vi "Cruft Dialog.vi"(11 "Path":path) -> (3 "Result":enum16{"Add", "Ignore", "Abort"}(ring))   [LabVIEW 2024]
panel:
  in  "Abort":bool
  out "Prompt":string
  in  "Ignore":bool
  in  "Add":bool
  out "Image":picture
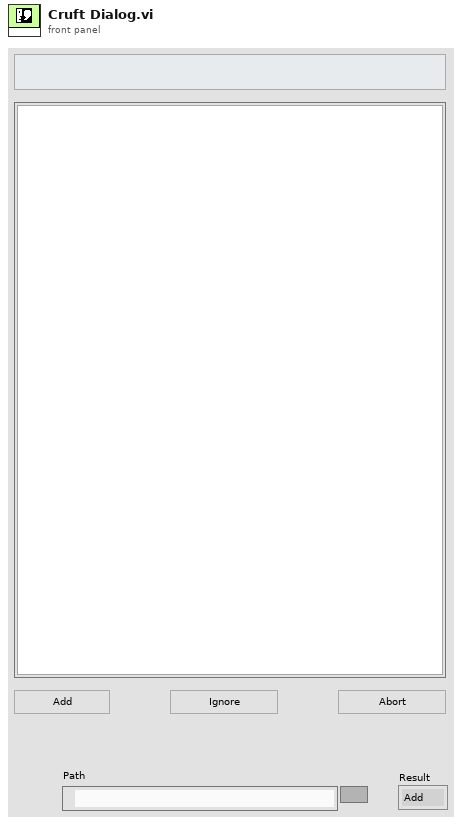
[diagram p1: front panel]
types:
  T1 = typedef "LVBoundsTypeDef.ctl" = cluster{"Width":u32, "Height":u32}
  T2 = typedef "imagedata.ctl" = cluster{"image type":i32, "image depth":i32, "image":u8[], "mask":u8[], "colors":u32[], "Rectangle":cluster{"left":i16, "top":i16, "right":i16, "bottom":i16}}
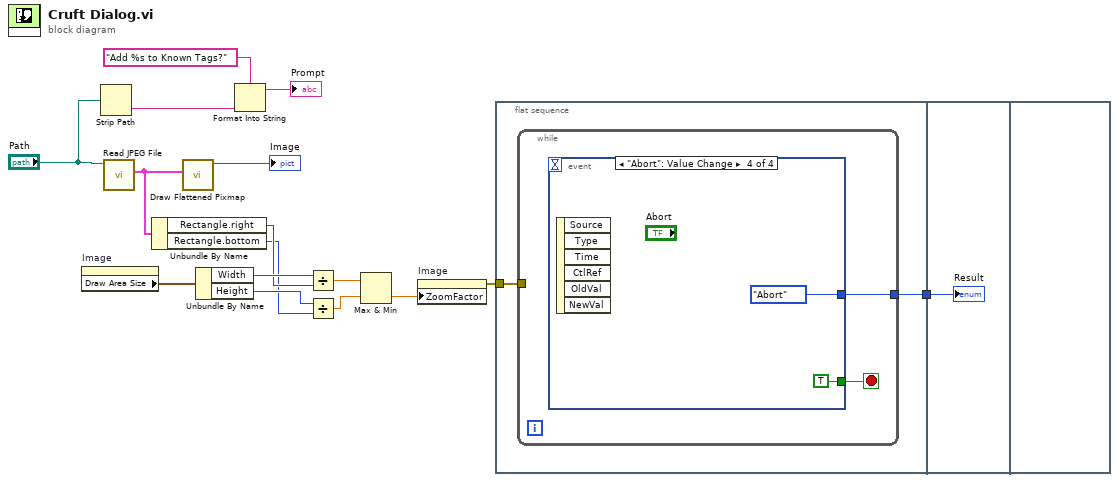
[diagram p0: block diagram]
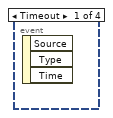
[diagram p2: hidden frame]
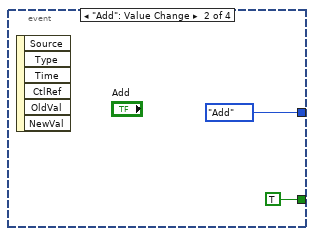
[diagram p3: hidden frame]
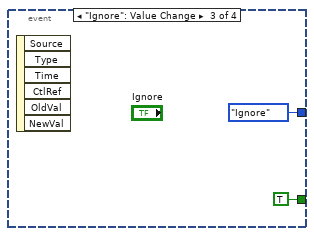
[diagram p4: hidden frame]
diagram:
  n1 = property on="Image" class="Pict"() -> ("Draw Area Size"=w15:T1)  [unwired: 2 in, 2 out]
  n2 = Strip Path(path="Path") -> (name=w3:string)  [unwired: 1 out]
  n3 = call <vilib>:"Read JPEG File.vi"("path to JPEG file"="Path") -> ("image data"=w14:T2)  [unwired: 8 in, 2 out]
  n4 = Unbundle By Name(w14) -> ("Rectangle.right"=w11:i16, "Rectangle.bottom"=w10:i16)
  n5 = call <vilib>:"Draw Flattened Pixmap.vi"("image data"=w14) -> ("new picture"=→"Image":picture)  [unwired: 8 in]
  n6 = Unbundle By Name(w15) -> ("Width"=w13:u32, "Height"=w12:u32)
  n7 = Format Into String(format string="Add %s to Known Tags?", w3) -> (resulting string=→"Prompt":string)  [unwired: 2 in, 1 out]
  n8 = Divide(x=w13, y=w11) -> (x/y=w9:dbl)
  n9 = Divide(x=w12, y=w10) -> (x/y=w8:dbl)
  n10 = Max & Min(x=w9, y=w8) -> (min(x,y)=w7:dbl)  [unwired: 1 out]
  n11 = property on="Image" class="Pict"("ZoomFactor"=w7) -> (error out=w6:errorcluster)  [unwired: 2 in, 1 out]
  n12 = flat-sequence {
    tunnel: w6 -> [w18]
    tunnel: [w17] -> w1
    tunnel: w1 -> [w27]
    frame #0 {
      n13 = while {
        tunnel: w18 -> [_]
        tunnel: [w20] -> w17
        stop <- w19 stop-if-true
        n14 = event shown="[3] \"Abort\": Value Change" {
          selector: _ -> [_ _ _ _]
          dyn-events: _ -> [_ _ _ _]
          timeout: _ -> [_ _ _ _]
          tunnel: [_ enum16{"Add", "Ignore", "Abort"}."Add" ("Result") enum16{"Add", "Ignore", "Abort"}."Ignore" ("Result") enum16{"Add", "Ignore", "Abort"}."Abort" ("Result")] -> w20
          tunnel: [_ TRUE TRUE TRUE] -> w19
          event Timeout {
            n15 = event-data() -> ()  [unwired: 1 in, 3 out]
          }
          event "Add": Value Change {
            n16 = event-data() -> ()  [unwired: 1 in, 6 out]
          }
          event "Ignore": Value Change {
            n17 = event-data() -> ()  [unwired: 1 in, 6 out]
          }
          event "Abort": Value Change {
            n18 = event-data() -> ()  [unwired: 1 in, 6 out]
          }
        }
      }
    }
    frame #1 {
      "Result" <- w27
    }
    frame #2 {
    }
  }
